vi "Define Element.vi"(8 "error in":errorcluster, 9 "Address":i32[](array[numeric]), 10 "Node Refnum":refnum<k20>) -> (0 "error out":errorcluster, 3 "Element out":refnum<class "Element.lvclass">)   [LabVIEW 2014, in "Element.lvclass"]
uses:
  Element.lvclass
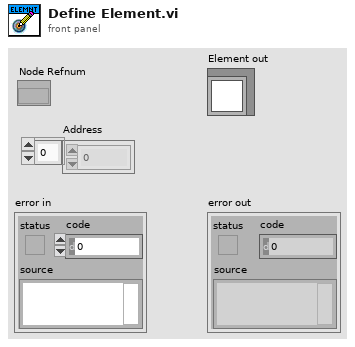
[diagram p1: front panel]
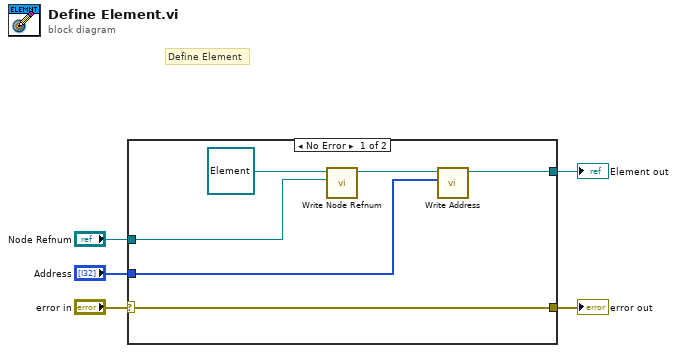
[diagram p0: block diagram]
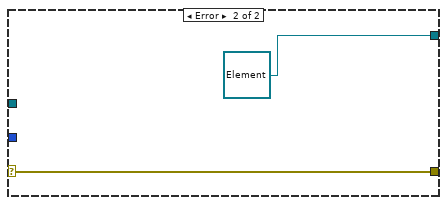
[diagram p2: hidden frame]
diagram:
  # "Define Element"
  n1 = case shown="No Error" "error in" {
    selector: "error in" -> [w11 w13]
    tunnel: [w11 w13] -> w4
    tunnel: [w7 refnum<class "Element.lvclass"> refnum ("Element.lvclass")] -> w3
    tunnel: "Node Refnum" -> [w8 _]
    tunnel: "Address" -> [w6 _]
    frame No Error {
      n2 = call-dynamic "Write Node Refnum.vi"("Node Refnum"=w8, "Node in"=refnum<class "Element.lvclass"> refnum ("Element.lvclass")) -> ("Node out"=w10:refnum<class "Element.lvclass">)  [unwired: 8 in, 1 out]
      n3 = call-dynamic "Write Address.vi"("Address"=w6, "Node in"=w10) -> ("Node out"=w7:refnum<class "Element.lvclass">)  [unwired: 8 in, 1 out]
    }
    frame Error {
    }
  }
  "error out" <- w4
  "Element out" <- w3
